vi "rp_wspr_geo1.vi"() -> ()   [LabVIEW 2014]
panel:
  in  "Path to Python.exe":path=path "C:/users/gregg/anaconda3/python.exe"
  out "standard output":string="mygs =  FN20\r\nband =  80m\r\ncallsign =  WB6YAZ\r\nantenna =  Longwire\r\ndmin =  180815.0\r\ndmax =  180815.0\r\ntmin =  0.0\r\ntmax =  2300.0\r\nnumber of datapoints = 503\r\nNumber of skipped datapoints = 0\r\nnumber of different locations = 1\r\n"
  out "error out 2":errorcluster
  out "standard error":string
  in  "antenna":string="Longwire"
  in  "tmax":string="2300"
  in  "tmin":string="0"
  in  "dmax":string="180816"
  in  "dmin":string="180815"
  in  "callsign":string="WB6YAZ"
  in  "band":string="80m"
  in  "mygs":string="FN20"
  # "Search Criteria"
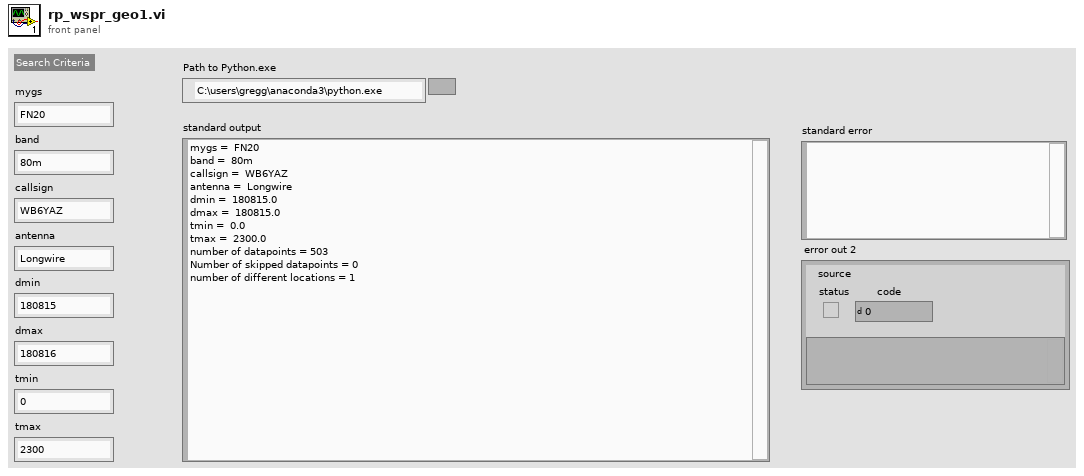
[diagram p1: front panel]
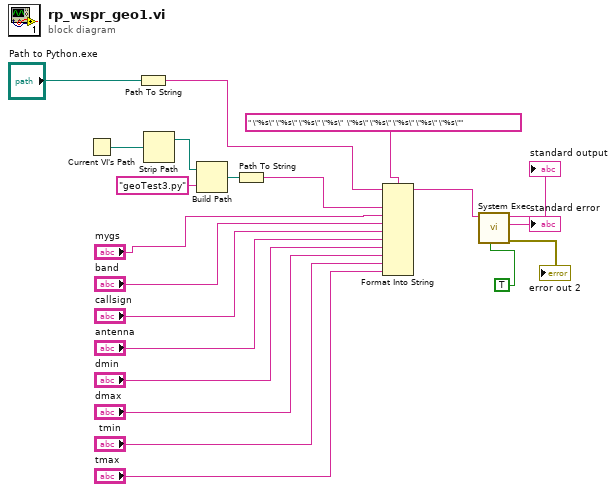
[diagram p0: block diagram]
diagram:
  n1 = Current VI's Path() -> (path=w18:path)
  n2 = Path To String(path="Path to Python.exe") -> (string=w3:string)
  n3 = Strip Path(path=w18) -> (stripped path=w17:path)  [unwired: 1 out]
  n4 = Build Path(base path=w17, name or relative path="geoTest3.py" ("Path to Function")) -> (appended path=w19:path)
  n5 = Path To String(path=w19) -> (string=w20:string)
  n6 = Format Into String(format string=" \"%s\" \"%s\" \"%s\" \"%s\"  \"%s\" \"%s\" \"%s\" \"%s\" \"%s\"", initial string=w3, w20, "mygs", "band", "callsign", "antenna", "dmin", "dmax", "tmin", "tmax") -> (resulting string=w7:string)  [unwired: 1 in, 1 out]
  n7 = call <vilib>:"System Exec.vi"("run minimized? (F)"=TRUE, "command line"=w7) -> ("error out"=→"error out 2":errorcluster, "standard error"=→"standard error":string, "standard output"=→"standard output":string)  [unwired: 6 in, 1 out]
